vi "Espinoza_Osorio_Salinas_Tipán_Labview Proyecto 1er Parcial.vi"() -> ()   [LabVIEW 2026]
uses:
  <vilib>/MakerHub/LINX/Public/Peripherals/Digital/Digital Read 1 Chan.vi
  <vilib>/MakerHub/LINX/Public/Peripherals/Analog/Analog Read 1 Chan.vi
  <vilib>/MakerHub/LINX/Public/Peripherals/Digital/Digital Read N Chans.vi
  <vilib>/MakerHub/LINX/Public/Peripherals/Analog/Analog Read N Chans.vi
  <vilib>/MakerHub/LINX/Private/Local IO/LinxDigitalRead.vi
  <vilib>/MakerHub/LINX/Public/Utilities/Check Channel.vi
  <vilib>/MakerHub/LINX/Private/Local IO/LinxAnalogRead.vi
  <vilib>/MakerHub/LINX/Public/Utilities/Open Serial.vi
  <vilib>/MakerHub/LINX/Private/Utilties/Generate Error.vi
  <vilib>/express/express shared/transition.llb/Dynamic To Waveform Array.vi
  <vilib>/express/express signal manip/GetorSetDDTAttributes/Set DDT Attributes/SetT0.vi
  <vilib>/express/express shared/transition.llb/Waveform Array To Dynamic.vi
  <vilib>/express/express signal manip/GetorSetDDTAttributes/Set DDT Attributes/Set DDT Properties.xnode
  <vilib>/express/express arith-compare/Formula/XNode/ExpressFormulaBlockNode.xnode
  <vilib>/MakerHub/LINX/LMH-LINX.lvlib
panel:
  out "ON/OFF":bool
  out "P3":bool
  out "P2":bool
  out "P1":bool
  out "LOW PRESSURE (RR)":bool
  out "LOW PRESSURE (RL)":bool
  out "LOW PRESSURE (FR)":bool
  out "LOW PRESSURE (FL)":bool
  out "VELOCIMETRO":dbl(knob) scale=0.0..240.0
  out "Oscilograma de Velocidad":dbl(graph)
  out "FL PSI":dbl
  out "PSI FR":dbl
  out "RR PSI":dbl
  out "RL PSI":dbl
  out "Velocidad kilometro/Hora":dbl
  out "Velocidad milla/hora":dbl
  out "RL bar":dbl
  out "RR bar":dbl
  out "FL bar":dbl
  out "BAR FR":dbl
  in  "Serial Port":refnum<visa-resource-name>="N/A"
  in  "stop":bool
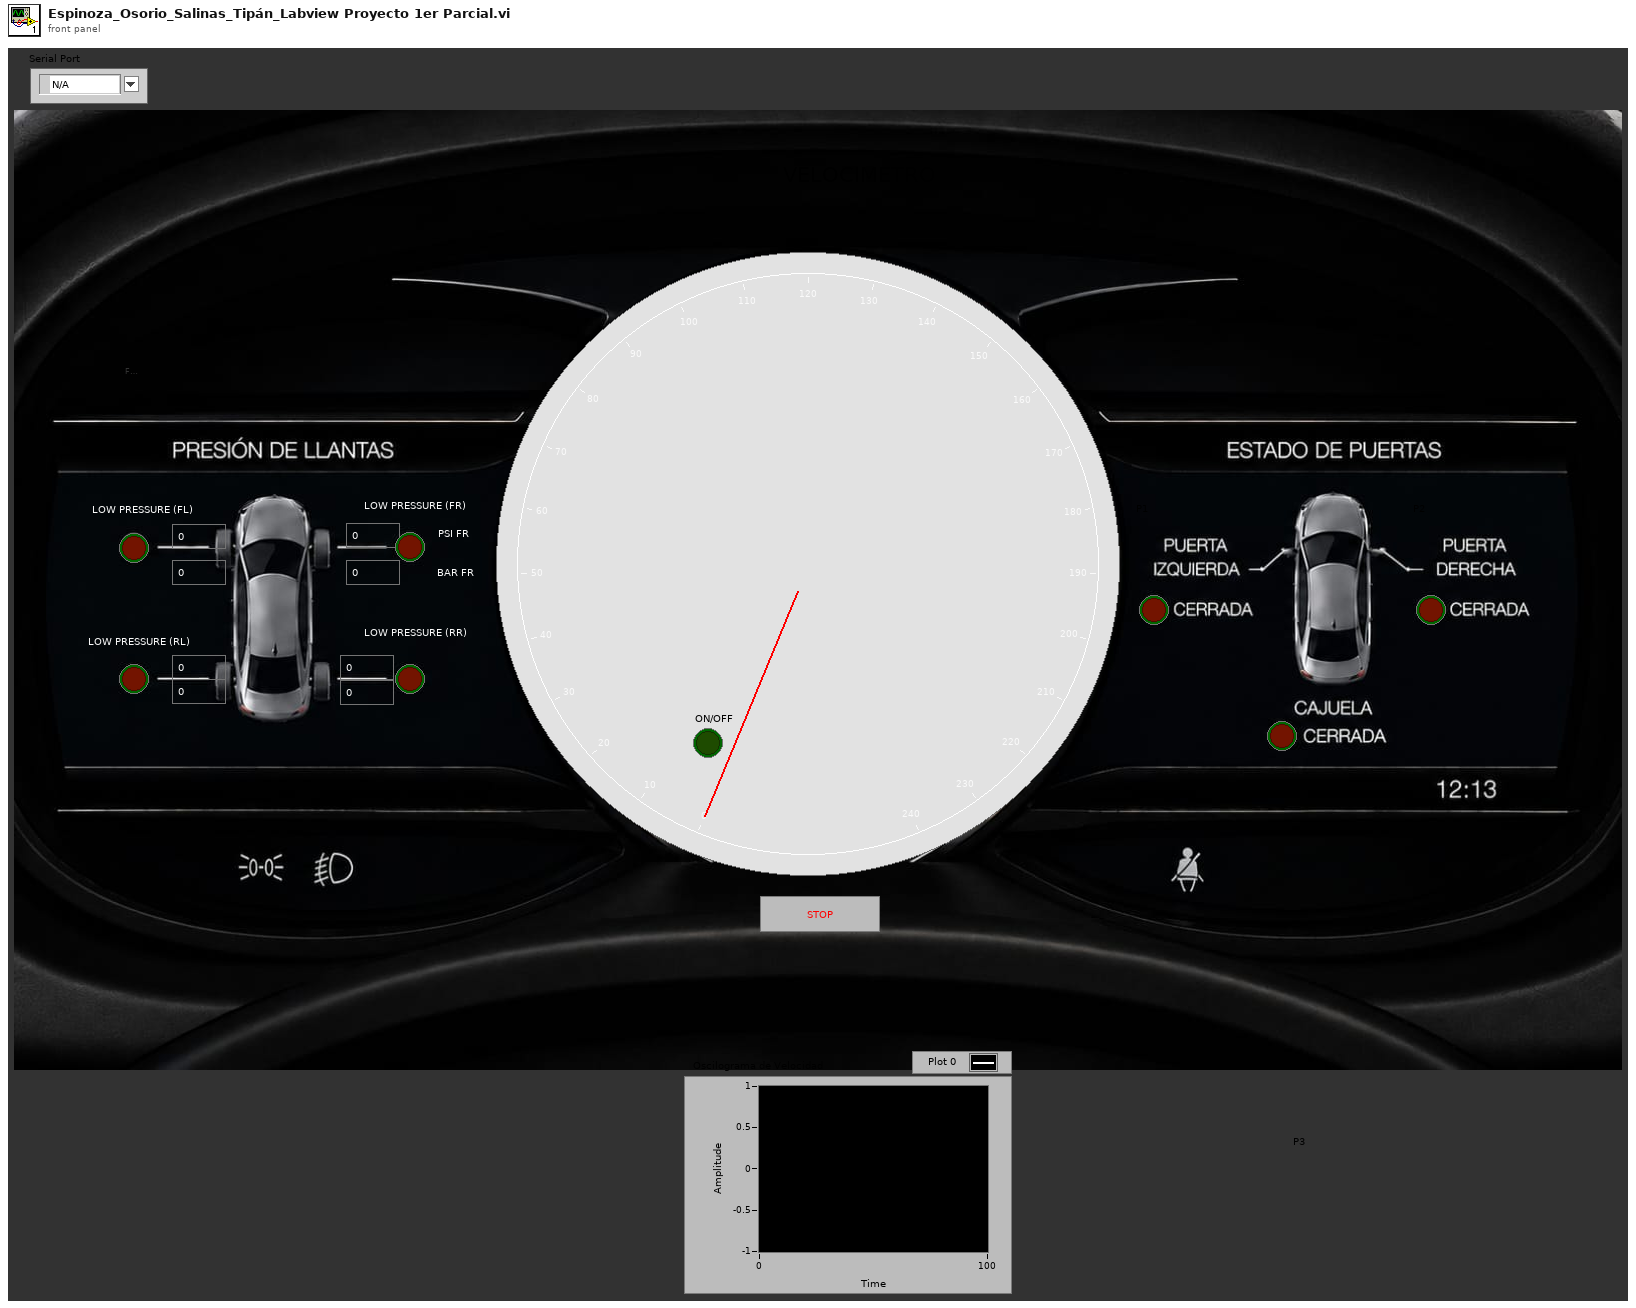
[diagram p1: front panel]
types:
  T1 = typedef "LMH-LINX.lvlib/LINX Ref.ctl" = cluster{"IO":T2, "Interface":T3, "LINX Device Config":T4}
  T2 = typedef "LMH-LINX.lvlib/Platform.ctl" = enum16{"Remote", "Local"}
  T3 = typedef "LMH-LINX.lvlib/Interface.ctl" = enum16{"Serial", "TCP"}
  T4 = typedef "LMH-LINX.lvlib/Device.lvlib/LINX Device Config.ctl" = cluster{"Interface":T3, "COM Port":refnum<visa-resource-name>, "TCP Configuration":T5, "Device Family":u8, "Device ID":u8, "Device Name":string, "TCP Ref":refnum<k5>, "Channels":T6}
  T5 = typedef "LMH-LINX.lvlib/Device.lvlib/TCP Config.ctl" = cluster{"IP Address":string, "Port":u16}
  T6 = typedef "LMH-LINX.lvlib/Channels.ctl" = cluster{"DI":u8[], "DO":u8[], "AI":u8[], "AO":u8[], "PWM":u8[], "QE":u8[], "UART":u8[], "I2C 2":u8[], "SPI":u8[], "CAN":u8[], "Servo":u8[], "AI Ref (V)":dbl, "AI Resolution (Bits)":u8, "AO Ref (V)":dbl, "AO Resolution (Bits)":u8}
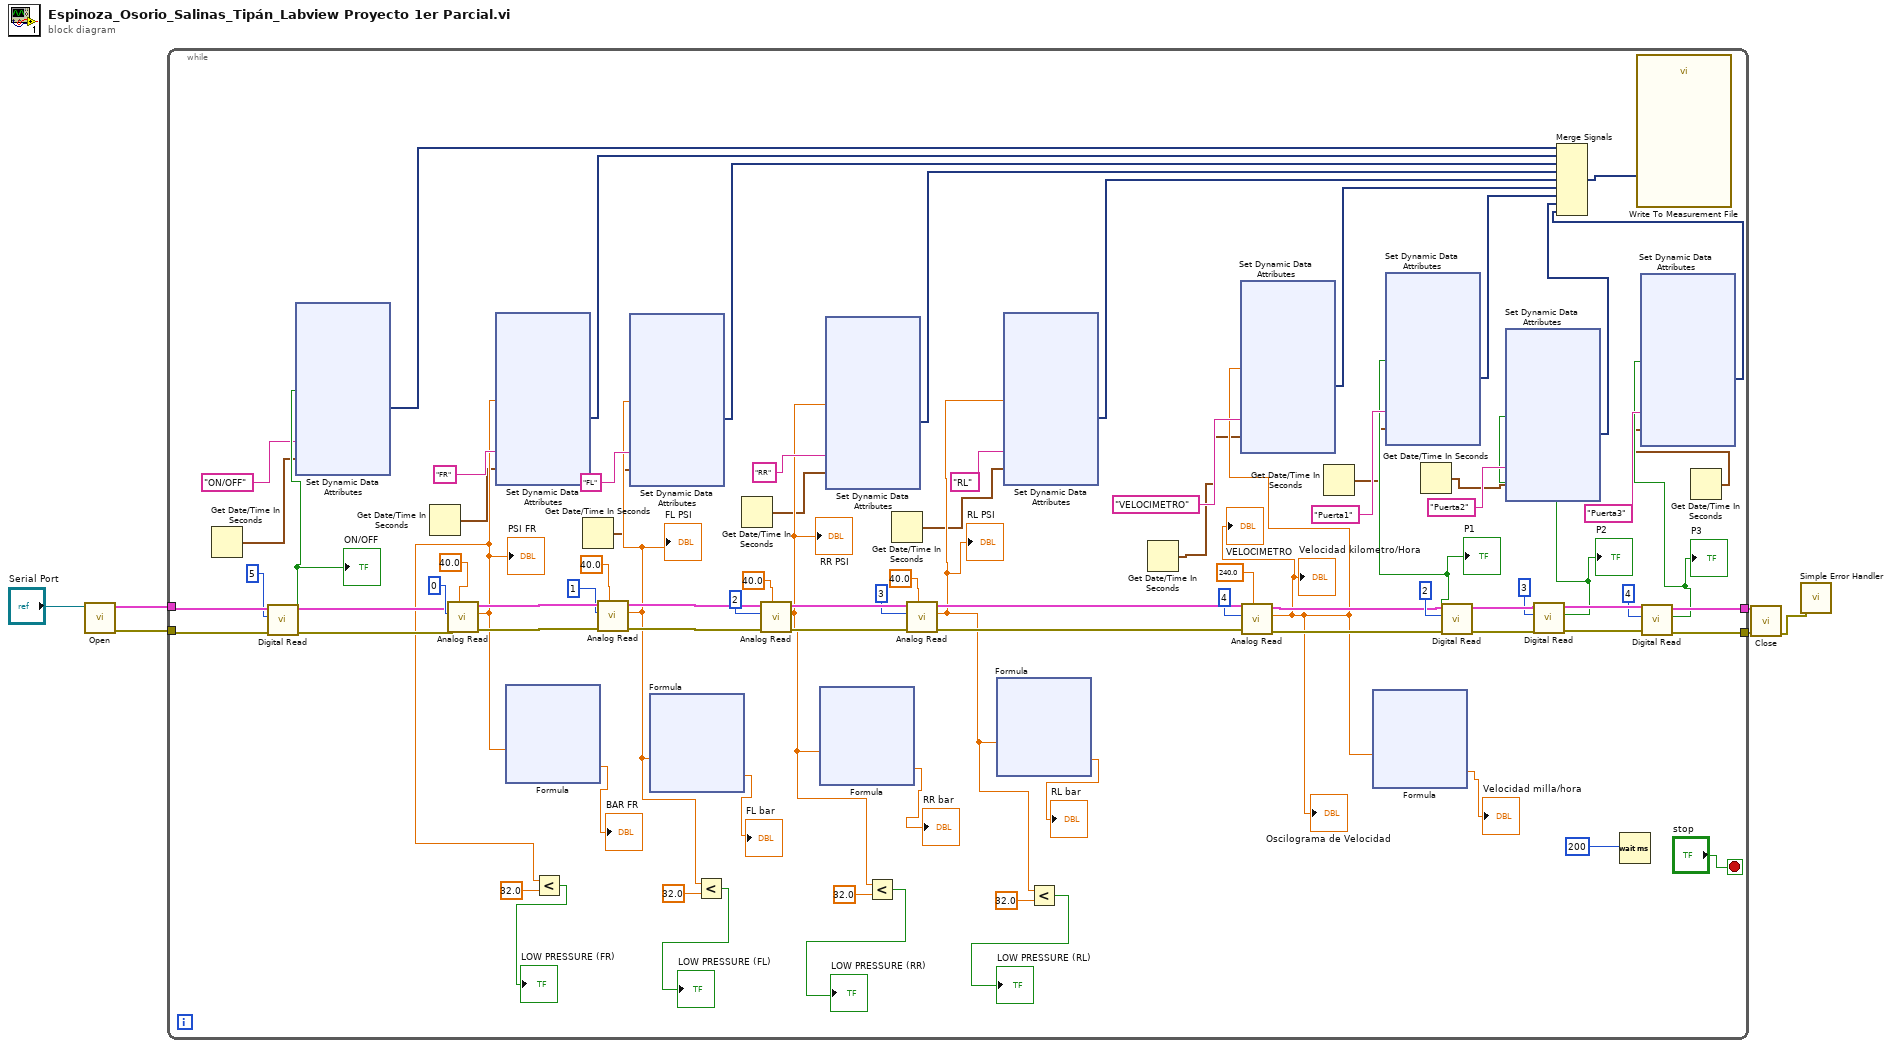
[diagram p0: block diagram]
diagram:
  n1 = call-poly <vilib>:"Open.vi"("Serial Port"="Serial Port") -> ("Error Out"=w3:errorcluster, "LINX Resource"=w4:T1)  [unwired: 8 in, 1 out]
  n2 = while {
    tunnel: w4 -> [w41]
    tunnel: w3 -> [w39]
    tunnel: [w67] -> w2
    tunnel: [w66] -> w1
    stop <- "stop" stop-if-true
    n3 = Get Date/Time In Seconds() -> (seconds since 1Jan1904=w15:timestamp)
    n4 = call-poly <vilib>:"Digital Read.vi"("Error In"=w39, "DI Channel"=5, "LINX Resource"=w41) -> ("Error Out"=w38:errorcluster, "DI Value"=w17:bool, "LINX Resource"=w40:T1)  [unwired: 6 in]
    "ON/OFF" <- w17
    n5 = xnode "Set Dynamic Data Attributes"("Signals In"=w17, "Signal Name"="ON/OFF", "Timestamp"=w15) -> ("Signals Out"=w18:dynamicdata)  [unwired: 2 in, 1 out]
    n6 = Get Date/Time In Seconds() -> (seconds since 1Jan1904=w14:timestamp)
    n7 = call-poly <vilib>:"Analog Read.vi"("Analog Ref Override (V)"=40.0, "Error In"=w38, "Analog Channel"=0, "LINX Resource"=w40) -> ("Error Out"=w91:errorcluster, "Voltage"=w32:dbl, "LINX Resource"=w92:T1)  [unwired: 4 in, 1 out]
    "PSI FR" <- w32
    n8 = xnode "Set Dynamic Data Attributes"("Signals In"=w32, "Signal Name"="FR", "Timestamp"=w14) -> ("Signals Out"=w36:dynamicdata)  [unwired: 2 in, 1 out]
    n9 = xnode "Formula"("X1"=w32) -> ("Result"=→"BAR FR":dbl)  [unwired: 1 in, 1 out]
    n10 = Less?(x=w32, y=32.0) -> (x < y?=→"LOW PRESSURE (FR)":bool)
    n11 = Get Date/Time In Seconds() -> (seconds since 1Jan1904=w13:timestamp)
    n12 = call-poly <vilib>:"Analog Read.vi"("Analog Ref Override (V)"=40.0, "Error In"=w91, "Analog Channel"=1, "LINX Resource"=w92) -> ("Error Out"=w89:errorcluster, "Voltage"=w27:dbl, "LINX Resource"=w90:T1)  [unwired: 4 in, 1 out]
    "FL PSI" <- w27
    n13 = xnode "Set Dynamic Data Attributes"("Signals In"=w27, "Signal Name"="FL", "Timestamp"=w13) -> ("Signals Out"=w54:dynamicdata)  [unwired: 2 in, 1 out]
    n14 = xnode "Formula"("X1"=w27) -> ("Result"=→"FL bar":dbl)  [unwired: 1 in, 1 out]
    n15 = Less?(x=w27, y=32.0) -> (x < y?=→"LOW PRESSURE (FL)":bool)
    n16 = Get Date/Time In Seconds() -> (seconds since 1Jan1904=w12:timestamp)
    n17 = call-poly <vilib>:"Analog Read.vi"("Analog Ref Override (V)"=40.0, "Error In"=w89, "Analog Channel"=2, "LINX Resource"=w90) -> ("Error Out"=w87:errorcluster, "Voltage"=w26:dbl, "LINX Resource"=w88:T1)  [unwired: 4 in, 1 out]
    "RR PSI" <- w26
    n18 = xnode "Formula"("X1"=w26) -> ("Result"=→"RR bar":dbl)  [unwired: 1 in, 1 out]
    n19 = xnode "Set Dynamic Data Attributes"("Signals In"=w26, "Signal Name"="RR", "Timestamp"=w12) -> ("Signals Out"=w52:dynamicdata)  [unwired: 2 in, 1 out]
    n20 = Less?(x=w26, y=32.0) -> (x < y?=→"LOW PRESSURE (RR)":bool)
    n21 = Get Date/Time In Seconds() -> (seconds since 1Jan1904=w11:timestamp)
    n22 = call-poly <vilib>:"Analog Read.vi"("Analog Ref Override (V)"=40.0, "Error In"=w87, "Analog Channel"=3, "LINX Resource"=w88) -> ("Error Out"=w85:errorcluster, "Voltage"=w25:dbl, "LINX Resource"=w86:T1)  [unwired: 4 in, 1 out]
    "RL PSI" <- w25
    n23 = xnode "Formula"("X1"=w25) -> ("Result"=→"RL bar":dbl)  [unwired: 1 in, 1 out]
    n24 = xnode "Set Dynamic Data Attributes"("Signals In"=w25, "Signal Name"="RL", "Timestamp"=w11) -> ("Signals Out"=w50:dynamicdata)  [unwired: 2 in, 1 out]
    n25 = Less?(x=w25, y=32.0) -> (x < y?=→"LOW PRESSURE (RL)":bool)
    n26 = Get Date/Time In Seconds() -> (seconds since 1Jan1904=w10:timestamp)
    n27 = call-poly <vilib>:"Analog Read.vi"("Analog Ref Override (V)"=240.0, "Error In"=w85, "Analog Channel"=4, "LINX Resource"=w86) -> ("Error Out"=w72:errorcluster, "Voltage"=w35:dbl, "LINX Resource"=w57:T1)  [unwired: 4 in, 1 out]
    "Velocidad kilometro/Hora" <- w35
    "Oscilograma de Velocidad" <- w35
    "VELOCIMETRO" <- w35
    n28 = xnode "Set Dynamic Data Attributes"("Signals In"=w35, "Signal Name"="VELOCIMETRO", "Timestamp"=w10) -> ("Signals Out"=w42:dynamicdata)  [unwired: 2 in, 1 out]
    n29 = Get Date/Time In Seconds() -> (seconds since 1Jan1904=w9:timestamp)
    n30 = xnode "Formula"("X1"=w35) -> ("Result"=→"Velocidad milla/hora":dbl)  [unwired: 1 in, 1 out]
    n31 = Get Date/Time In Seconds() -> (seconds since 1Jan1904=w8:timestamp)
    n32 = call-poly <vilib>:"Digital Read.vi"("Error In"=w72, "DI Channel"=2, "LINX Resource"=w57) -> ("Error Out"=w70:errorcluster, "DI Value"=w21:bool, "LINX Resource"=w71:T1)  [unwired: 6 in]
    "P1" <- w21
    n33 = xnode "Set Dynamic Data Attributes"("Signals In"=w21, "Signal Name"="Puerta1", "Timestamp"=w9) -> ("Signals Out"=w48:dynamicdata)  [unwired: 2 in, 1 out]
    n34 = call-poly <vilib>:"Digital Read.vi"("Error In"=w70, "DI Channel"=3, "LINX Resource"=w71) -> ("Error Out"=w68:errorcluster, "DI Value"=w20:bool, "LINX Resource"=w69:T1)  [unwired: 6 in]
    "P2" <- w20
    n35 = xnode "Set Dynamic Data Attributes"("Signals In"=w20, "Signal Name"="Puerta2", "Timestamp"=w8) -> ("Signals Out"=w47:dynamicdata)  [unwired: 2 in, 1 out]
    n36 = Wait (ms)(milliseconds to wait=u32 200 ("millisecond timer value")) -> ()  [unwired: 1 out]
    n37 = call-poly <vilib>:"Digital Read.vi"("Error In"=w68, "DI Channel"=4, "LINX Resource"=w69) -> ("Error Out"=w67:errorcluster, "DI Value"=w19:bool, "LINX Resource"=w66:T1)  [unwired: 6 in]
    "P3" <- w19
    n38 = Get Date/Time In Seconds() -> (seconds since 1Jan1904=w7:timestamp)
    n39 = xnode "Set Dynamic Data Attributes"("Signals In"=w19, "Signal Name"="Puerta3", "Timestamp"=w7) -> ("Signals Out"=w46:dynamicdata)  [unwired: 2 in, 1 out]
    n40 = Merge Signals(w18, w36, w54, w52, w50, w42, w48, w47, w46) -> (w62:dynamicdata)
    n41 = call "Write To Measurement File"("Signals"=w62) -> ()  [unwired: 16 in, 3 out]
  }
  n42 = call <vilib>:"Close.vi"("Error In"=w2, "LINX Resource"=w1) -> ("Error Out"=w5:errorcluster)  [unwired: 9 in]
  n43 = call <vilib>:"Simple Error Handler.vi"("error in (no error)"=w5) -> ()  [unwired: 4 in, 5 out]
